vi "Set Current Limits.vi"(8 "error in (no error)":errorcluster, 10 "current_limits":dbl[](array[numeric]) min=0.0 max=0.9 step=0.01, 11 "MF3 in":refnum<class "MF3.lvclass">) -> (0 "error out":errorcluster, 3 "MF3 out":refnum<class "MF3.lvclass">)   [LabVIEW 2011, in "MF3.lvclass"]
uses:
  MF3.lvclass
  MF3.lvclass/MF3.ctl
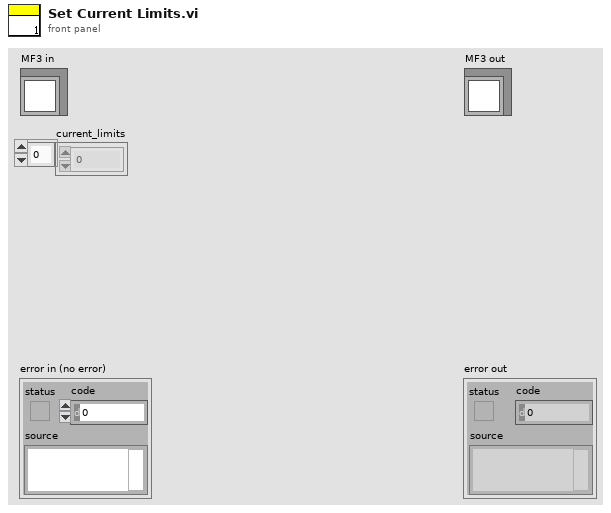
[diagram p1: front panel]
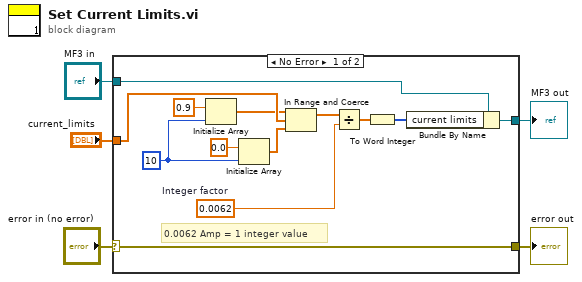
[diagram p0: block diagram]
diagram:
  n1 = case shown="No Error" "error in (no error)" {
    selector: "error in (no error)" -> [w9 w20]
    tunnel: [w9 w20] -> w4
    tunnel: [w6 w19] -> w2
    tunnel: "MF3 in" -> [w8 w19]
    tunnel: "current_limits" -> [w16 _]
    frame No Error {
      w12 = 10 ("dimension size")
      w18 = 0.0062  # Integer factor
      # "0.0062 Amp = 1 integer value"
      n2 = Initialize Array(0.9 ("element"), w12) -> (w14:dbl[])
      n3 = Initialize Array(0.0 ("element"), w12) -> (w11:dbl[])
      n4 = In Range and Coerce(upper limit=w14, x=w16, lower limit=w11) -> (coerced(x)=w10:dbl[])  [unwired: 1 out]
      n5 = Divide(x=w10, y=w18) -> (x/y=w17:dbl[])
      n6 = To Word Integer(number=w17) -> (16bit integer=w7:i16[])
      n7 = Bundle By Name(cluster=w8, "current limits"=w7) -> (w6:refnum<class "MF3.lvclass">)
    }
    frame Error {
    }
  }
  "error out" <- w4
  "MF3 out" <- w2
